vi "Main_08a.vi"() -> ()   [LabVIEW 2023]
uses:
  Map_Direction.ctl
  Cluster_Right Left.ctl
  <vilib>/Utility/error.llb/Trim Whitespace One-Sided.vi
panel:
  out "Map":T1
  in  "Example 2":string="LLR\n\nAAA = (BBB, BBB)\nBBB = (AAA, ZZZ)\nZZZ = (ZZZ, ZZZ)"
  out "Answer":i32
  in  "Puzzle":string="LRRLRRLRRRLRLLRRRLLRRRLRLRRRLRLRRLRRRLRRRLRLRRRLRRRLRRLRRRLLLRLRRRLRRRLRRRLRLRLRRLLRRRLRLLRLRRRLRRLLRLRLRRLRRRLRRLLRLRRRLLRRLRRRLRLRRLLRRRLRRLLRRLRRRLRLRRRLRRLRRRLRRRLRRLRRRLRLRRLRRRLRRRLRRLLRLRRLRRLRRRLRLLLRRRLLRRRLRLRRRLRLRRLRRRLLLRLRRRLRLRRLRRRLRRRLRRLRLRLRRRR\n\nPBN = (JRP, RVT)\nXRS = (CRH, SXK)\nMLN = (STJ, MGB)\nXGX = (XGM, GKP)\nVDC = (DBF, FVR)\nNBC = (QQJ, XKG)\nKRC = (QVQ, RJL)\nLCX = (CSN, DBP)\nMSX = (LVF, PPD)\nMMF = (GBX, LCX)\nBXQ = (MPS, GLM)\nGTL = (VSF, DVZ)\nSVR = (FKK, FJN)\nHJJ = (XPS, HVS)\nMHL = (HTN, HTG)\nLGQ = (NJT, NML)\nKFR = (TXK, DHG)\nMXQ = (DGJ, MKP)\nXST = (MGP, QSK)\nBNJ = (NBC, DFB)\nJLK = (RJS, XDM)\nBKS = (SLF, PLK)\nLCV = (RVB, CJV)\nGJL = (FRB, QNK)\nFPD = (SFN, MLS)\nHMJ = (MXK, CRR)\nSQF = (MCC, QXB)\nCGC = (SCS, FFB)\nCTP = (RJQ, BSV)\nQCF = (JCB, TKP)\nLBJ = (XKV, DQM)\nRMC = (LLD, TTP)\nLHK = (CDB, TSV)\nHPC = (QLX, QPQ)\nVXC = (PLF, SSV)\nRDT = (GJL, TTN)\nSDB = (MVL, FRF)\nHRT = (DVS, BHX)\nMHR = (VXR, VQN)\nRPT = (BLP, DDP)\nJFF = (DCJ, XST)\nNDL = (NJQ, BNC)\nFXL = (MSC, JSR)\nDVZ = (JVJ, KLP)\nXGD = (RFH, DTL)\nMPR = (QNN, CKH)\nSBB = (VTK, TSS)\nDRJ = (GHM, NFK)\nLXL = (SSJ, CQR)\nBTN = (MXN, HLF)\nSMX = (VFT, NKJ)\nRJQ = (STS, GLR)\nQLV = (PNP, TDK)\nQMJ = (MKP, DGJ)\nXDM = (SFB, JLN)\nLFX = (CDM, LMX)\nQTX = (RVB, CJV)\nCPX = (TTH, CBK)\nTFF = (CLG, LGN)\nJDC = (BHH, HFJ)\nTXV = (JVF, FXS)\nLBP = (PRS, PRS)\nLND = (QLV, TLK)\nRXR = (BVT, QKX)\nRSR = (GFN, GVL)\nFLG = (RMC, LTD)\nTPB = (PJP, QCL)\nKQH = (LRG, MRL)\nVVN = (KPP, HJH)\nNTR = (RPQ, GFG)\nQDK = (JFC, XGN)\nVBA = (KLP, JVJ)\nXSP = (KVF, VJV)\nHVB = (CQR, SSJ)\nXBN = (GBD, TCS)\nRFH = (FGN, NSP)\nHTN = (NBH, SMP)\nPSD = (FLS, KCJ)\nMGB = (SDF, MHR)\nNXT = (HKQ, MLD)\nMHC = (JSR, MSC)\nKPP = (HHV, FNC)\nTSS = (RBD, LGQ)\nBMS = (NLL, NFJ)\nBKV = (NLK, BBH)\nSDF = (VXR, VQN)\nGLR = (LFX, XXL)\nNBN = (SXB, DLD)\nCVV = (KGX, DTQ)\nVKG = (VNG, PTR)\nFJR = (KNQ, XGX)\nRJN = (PGR, QCV)\nCNJ = (LSV, BVN)\nDTC = (RXR, MHX)\nFVB = (BSM, BGR)\nSFG = (KSP, GXM)\nPLN = (PDV, XJD)\nTHL = (KRC, HXH)\nPNP = (JQQ, SMV)\nSTS = (LFX, XXL)\nNNC = (MPG, RVG)\nNJT = (JGJ, CGH)\nSCS = (NSR, DXX)\nGSF = (LHP, FTK)\nGBD = (DSN, HRT)\nJVF = (HPT, QHF)\nPSV = (NJC, CPH)\nJLP = (FGD, BFF)\nCRR = (PRB, HCH)\nFVJ = (VBP, BBQ)\nMVL = (CGS, BFN)\nJXK = (SFN, MLS)\nSSV = (DJB, TRK)\nLXQ = (LSB, SPC)\nLHS = (SSV, PLF)\nDDK = (QXR, QCF)\nXKG = (BTS, KFL)\nTSM = (QCV, PGR)\nCPT = (TMH, DFQ)\nDGJ = (MMD, PJN)\nMQP = (CFG, LRB)\nRQM = (JTK, PLN)\nPLK = (KQF, HSZ)\nHVC = (NLK, BBH)\nLSB = (NDT, TPG)\nRMN = (SKJ, PBH)\nQXL = (JNC, XMH)\nTDD = (BSX, GBR)\nBGP = (LBP, LBP)\nTVA = (FBB, VBN)\nVSB = (VNG, PTR)\nXLH = (HMX, FJX)\nNVQ = (RPQ, RPQ)\nFMN = (BSV, RJQ)\nXMC = (QCD, RJK)\nHPT = (HGL, GNS)\nCMS = (KVT, FQR)\nQHF = (HGL, GNS)\nQNT = (BPT, FLG)\nKVD = (SLL, GGK)\nDMK = (HKT, CGD)\nCRM = (BTR, GHV)\nTPJ = (GCT, DQD)\nKFL = (RDG, VDC)\nQCR = (DNK, THD)\nCLV = (MTS, PBN)\nZZZ = (DPM, TCG)\nQHN = (TNC, KVD)\nNRP = (SQL, PMR)\nJNH = (TKD, LQF)\nVPR = (PKX, CTD)\nLVD = (MQC, QKJ)\nXRM = (BRM, MPR)\nFFB = (NSR, DXX)\nMGR = (MNB, TSP)\nFMK = (THR, VGR)\nKVT = (GSN, RXF)\nVMS = (LPM, VJP)\nDVA = (MHC, FXL)\nMXS = (RJS, XDM)\nKXV = (KPF, NKX)\nBBH = (XSP, GMD)\nPKX = (XHC, CPV)\nNSL = (SMX, DNM)\nDXV = (LPM, VJP)\nCCC = (LCX, GBX)\nJVS = (HJJ, FLF)\nHPM = (QSF, CPT)\nFVS = (XXR, CGF)\nPPB = (XGX, KNQ)\nXPF = (SMX, DNM)\nHLF = (NQJ, CVV)\nTJS = (LXQ, VFB)\nFJK = (FGD, BFF)\nQGQ = (FVJ, BDV)\nGRR = (JKM, JLH)\nGHV = (XGD, QBH)\nRVT = (PVB, PCS)\nTBL = (VGK, KTT)\nSNR = (GCT, DQD)\nXSK = (BLL, MNF)\nVDS = (CCC, MMF)\nRVG = (XSK, XSJ)\nTKP = (MLN, KRX)\nSRP = (QLV, TLK)\nFXQ = (LVD, RHD)\nLVC = (LCT, LKS)\nHNC = (MQP, KTG)\nDFP = (NMX, JFX)\nJVT = (SNX, KQK)\nJSR = (KXN, LXS)\nHCV = (MFD, KJX)\nRBJ = (JKT, HLZ)\nHFC = (JFX, NMX)\nXQG = (PGD, XFT)\nFRB = (HCP, LVJ)\nLQF = (QCR, XTL)\nVGR = (RMN, LNQ)\nMMN = (HDR, JTL)\nPJN = (VNM, KHQ)\nTRK = (NSL, XPF)\nTVG = (CJH, THL)\nDMH = (GPM, MSX)\nVTK = (RBD, LGQ)\nTMH = (BSQ, CMT)\nJPN = (LTH, LST)\nSFB = (NKN, RFM)\nCGD = (VBH, ZZZ)\nVNM = (LMT, VRQ)\nNNT = (HHX, NTF)\nVFQ = (HMJ, VFV)\nSQL = (BCQ, NBN)\nQKJ = (GHN, HCK)\nMMR = (KMF, HPM)\nPFS = (HVL, CTG)\nFVD = (LBJ, DVM)\nSLF = (KQF, KQF)\nBBQ = (RSV, LHK)\nTCG = (NGG, LLS)\nBLR = (PTL, MSR)\nCVH = (MVL, FRF)\nGHN = (CKF, HTV)\nXQC = (QXR, QCF)\nGCT = (BGP, BGP)\nXMJ = (BVN, LSV)\nLBH = (VQX, SBC)\nBNC = (LNH, CRM)\nTHP = (KBC, MHH)\nVRQ = (VVN, THX)\nBFN = (SGD, QXL)\nTFH = (TDD, HGV)\nMLS = (PRJ, JPQ)\nXDQ = (BXQ, RQR)\nDJS = (MTS, PBN)\nSSK = (HKQ, MLD)\nVBH = (TCG, DPM)\nNNJ = (JHS, KFR)\nJRP = (PCS, PVB)\nFDK = (SRP, LND)\nFCL = (HPC, NGH)\nBGR = (MFV, CXJ)\nHDR = (FXQ, KSN)\nPPD = (PKL, KTR)\nBLP = (DKJ, DKJ)\nBCX = (PTL, MSR)\nFLF = (HVS, XPS)\nJPQ = (DMH, RTN)\nGNS = (SLT, HHM)\nGVH = (PRS, XKZ)\nPDV = (VDK, VDK)\nPQF = (BQN, CHK)\nSCX = (NLL, NFJ)\nJNC = (VNN, FVD)\nTHR = (LNQ, RMN)\nVBP = (RSV, LHK)\nMTS = (JRP, RVT)\nNKG = (RPG, TFH)\nLXK = (JXM, GSF)\nTXK = (RJC, QNT)\nSMV = (FTJ, GPD)\nDCP = (FFB, SCS)\nCJK = (FJR, PPB)\nLGN = (NLF, MTJ)\nCKF = (SMF, BSH)\nTRP = (TNC, KVD)\nTPG = (DJM, XMK)\nVJC = (JSX, NBT)\nLFK = (RXR, MHX)\nSBX = (FJN, FKK)\nFBB = (BMS, SCX)\nBHX = (SDN, HTF)\nCSN = (NHV, QVH)\nQQJ = (BTS, KFL)\nHFJ = (MMR, KCR)\nSVS = (GFN, GVL)\nFJL = (CJJ, GQF)\nDHG = (QNT, RJC)\nPCS = (VFG, SQF)\nRVB = (SBB, TND)\nPVB = (SQF, VFG)\nLPJ = (LRK, LXK)\nGVL = (NGL, GNV)\nCTJ = (QCD, RJK)\nPQB = (HMD, TQB)\nMCC = (SFV, DVV)\nQXX = (VBC, QGQ)\nRNM = (XXQ, LLT)\nHXB = (TRP, QHN)\nJFC = (TFF, DFC)\nSQQ = (JQL, HNC)\nKHQ = (LMT, VRQ)\nXCC = (FMK, DGK)\nJTL = (FXQ, KSN)\nNLF = (MLK, PLD)\nFVR = (GVK, CMS)\nSMF = (SNR, TPJ)\nNJL = (TRP, QHN)\nCSR = (DVP, KHX)\nQNJ = (THL, CJH)\nSBT = (XST, DCJ)\nRLX = (DGK, FMK)\nTHX = (KPP, HJH)\nKTG = (CFG, LRB)\nPVC = (RQR, BXQ)\nDLD = (GSM, DTT)\nBFF = (JBH, JVT)\nQKX = (FQJ, SFJ)\nDQD = (BGP, XHS)\nVFB = (LSB, SPC)\nMSR = (VBK, JTQ)\nCKB = (HHX, NTF)\nFLS = (QNM, PQB)\nQSF = (TMH, DFQ)\nFTK = (FDK, FLQ)\nFJX = (JVC, GXS)\nBDF = (MPR, BRM)\nMXK = (PRB, HCH)\nSDQ = (FJX, HMX)\nJCC = (TSP, MNB)\nGKP = (JLK, MXS)\nMRL = (FVS, NLQ)\nDPM = (LLS, NGG)\nGFL = (DDJ, NKG)\nFBG = (RDT, MVG)\nKJX = (VCJ, GHB)\nGFC = (LLT, XXQ)\nLVJ = (DJS, CLV)\nKNQ = (XGM, GKP)\nNJN = (FLS, KCJ)\nDSS = (KPF, NKX)\nJVC = (FHD, BMQ)\nTVP = (TBL, MVX)\nBQN = (SHT, TPS)\nDFQ = (CMT, BSQ)\nGXS = (FHD, BMQ)\nLRK = (JXM, GSF)\nKGX = (NDL, XDN)\nVTD = (SXK, CRH)\nKHH = (HKT, HKT)\nNTF = (NVQ, NTR)\nKRX = (STJ, MGB)\nSPC = (NDT, TPG)\nDJM = (JPN, TNG)\nTHD = (VFQ, GCC)\nCLG = (NLF, MTJ)\nNKN = (SRT, VHH)\nGGK = (RLX, XCC)\nHHV = (LCV, QTX)\nLRG = (NLQ, FVS)\nGNG = (BDF, XRM)\nFNC = (QTX, LCV)\nMVV = (QDK, LNK)\nQTH = (MSH, XDC)\nMKP = (MMD, PJN)\nVBC = (FVJ, BDV)\nJKT = (FJL, BNB)\nMFV = (SVS, RSR)\nHKX = (CPH, NJC)\nHCH = (BKV, HVC)\nTLK = (TDK, PNP)\nDNK = (GCC, VFQ)\nVXR = (NJV, KLH)\nMPG = (XSJ, XSK)\nJLN = (NKN, RFM)\nLTH = (QQS, TXV)\nFLQ = (LND, SRP)\nSXN = (MHL, MHL)\nCFG = (BXX, NRP)\nNDT = (XMK, DJM)\nTTP = (VPX, SXR)\nQXR = (TKP, JCB)\nTDK = (JQQ, SMV)\nKXN = (NXH, BNJ)\nVPA = (HTN, HTG)\nVHH = (DSG, NCN)\nAAA = (TCG, DPM)\nGHM = (NNC, VKX)\nGPM = (PPD, LVF)\nCGH = (LVC, BMH)\nNJQ = (LNH, CRM)\nDKB = (HPC, NGH)\nVKB = (KBC, MHH)\nCKH = (LXL, HVB)\nTSP = (BNN, CBJ)\nFKS = (JTK, PLN)\nNGH = (QLX, QPQ)\nMFT = (QMR, CDQ)\nBSV = (GLR, STS)\nRQR = (GLM, MPS)\nDDP = (DKJ, GTL)\nSQP = (MVG, RDT)\nLMX = (PLH, DDV)\nJCB = (KRX, MLN)\nHCP = (DJS, CLV)\nKQF = (MHC, FXL)\nNML = (CGH, JGJ)\nDRG = (KFR, JHS)\nNLQ = (XXR, CGF)\nBNB = (CJJ, GQF)\nMNF = (SQH, HCV)\nHTF = (FHL, FTC)\nJKM = (QNJ, TVG)\nCDM = (DDV, PLH)\nJHS = (TXK, DHG)\nBDK = (TTH, CBK)\nQVQ = (XJC, MFT)\nMMD = (VNM, KHQ)\nRFC = (HVL, CTG)\nBNN = (FGS, SFG)\nQCL = (GFL, KKH)\nKSN = (RHD, LVD)\nXMN = (XQC, DDK)\nNJC = (TSM, RJN)\nSQH = (MFD, KJX)\nQCD = (KHH, KHH)\nKTT = (PSV, HKX)\nSRT = (NCN, DSG)\nMHX = (QKX, BVT)\nCBJ = (FGS, SFG)\nTTH = (TMF, FPL)\nDBF = (GVK, CMS)\nDNM = (NKJ, VFT)\nXGM = (MXS, JLK)\nNLL = (FMJ, CPM)\nHMD = (FKS, RQM)\nPXT = (JTL, HDR)\nGHB = (GGQ, MVV)\nQCV = (VMS, DXV)\nSBC = (FJK, JLP)\nSGD = (XMH, JNC)\nJQQ = (FTJ, GPD)\nJLH = (TVG, QNJ)\nKPF = (XDQ, PVC)\nVQX = (JLP, FJK)\nVDK = (SLF, SLF)\nPLH = (SBX, SVR)\nQNN = (LXL, HVB)\nSXB = (GSM, DTT)\nJQL = (MQP, KTG)\nJXM = (LHP, FTK)\nQXB = (SFV, DVV)\nVBK = (BDK, CPX)\nBVT = (FQJ, SFJ)\nBHK = (KXV, DSS)\nCJJ = (MXQ, QMJ)\nXTL = (DNK, THD)\nBDV = (BBQ, VBP)\nCPH = (RJN, TSM)\nDTA = (FJL, BNB)\nTQB = (FKS, RQM)\nKMR = (NNT, CKB)\nLRB = (BXX, NRP)\nMVG = (TTN, GJL)\nXXL = (LMX, CDM)\nLMT = (VVN, THX)\nQMR = (PFS, RFC)\nBKD = (DVP, KHX)\nQNK = (LVJ, HCP)\nDGK = (THR, VGR)\nXHC = (FBG, SQP)\nTNC = (GGK, SLL)\nVJP = (GGM, HJD)\nVQN = (NJV, KLH)\nLLD = (SXR, VPX)\nXDC = (CST, BHK)\nKQK = (CNJ, XMJ)\nXJC = (QMR, CDQ)\nKKH = (NKG, DDJ)\nFRF = (CGS, BFN)\nFGS = (KSP, GXM)\nGSB = (GBK, VDS)\nNKX = (XDQ, PVC)\nSDN = (FHL, FTC)\nBVN = (CTP, FMN)\nQSK = (DCB, KSC)\nCTD = (CPV, XHC)\nNBH = (XBN, NVB)\nHRS = (LGD, VSK)\nJTQ = (CPX, BDK)\nCMT = (HXP, KMR)\nDKJ = (VSF, VSF)\nVNG = (KQH, PCC)\nCPV = (SQP, FBG)\nNBT = (HJK, GNG)\nVCJ = (GGQ, MVV)\nLNQ = (SKJ, PBH)\nDFB = (QQJ, XKG)\nRJC = (FLG, BPT)\nSFV = (XMN, QJS)\nRHD = (MQC, QKJ)\nQQS = (JVF, FXS)\nNHV = (BMN, GRR)\nNGG = (SQQ, CQQ)\nXGN = (TFF, DFC)\nHCK = (CKF, HTV)\nSNX = (CNJ, XMJ)\nPRB = (HVC, BKV)\nSXR = (SSK, NXT)\nGGQ = (LNK, QDK)\nDCJ = (QSK, MGP)\nMFD = (GHB, VCJ)\nGLM = (XQG, PDF)\nTND = (TSS, VTK)\nJFB = (BLP, BLP)\nKSC = (VKB, THP)\nCXJ = (SVS, RSR)\nVMT = (MXN, HLF)\nNSP = (HCC, TVP)\nBSK = (PKX, CTD)\nMPS = (XQG, PDF)\nNJV = (CJK, MKD)\nCGF = (CGC, DCP)\nGMD = (VJV, KVF)\nCRL = (PJP, QCL)\nMGP = (KSC, DCB)\nCQQ = (JQL, HNC)\nGGZ = (HTG, HTN)\nTNG = (LST, LTH)\nCST = (KXV, DSS)\nVFV = (CRR, MXK)\nRPG = (TDD, HGV)\nCQR = (DRG, NNJ)\nKSP = (DPT, GSB)\nVKX = (MPG, RVG)\nFMJ = (PQF, CVL)\nSLL = (RLX, XCC)\nHLZ = (BNB, FJL)\nGXM = (GSB, DPT)\nBSH = (SNR, TPJ)\nHGL = (HHM, SLT)\nQVH = (GRR, BMN)\nBTR = (XGD, QBH)\nRBD = (NML, NJT)\nHXP = (NNT, CKB)\nBMP = (JCC, MGR)\nKLP = (FGF, TJS)\nNRK = (VBC, QGQ)\nXMK = (TNG, JPN)\nPBH = (GCL, LPJ)\nNSR = (JFB, RPT)\nSHT = (JVS, HKN)\nNVB = (GBD, TCS)\nMLK = (QTH, GTT)\nFTC = (BSK, VPR)\nPCC = (MRL, LRG)\nPTL = (VBK, JTQ)\nNKJ = (FCL, DKB)\nGFN = (NGL, NGL)\nMQC = (GHN, HCK)\nKMF = (QSF, CPT)\nDDV = (SBX, SVR)\nKHX = (BLR, BCX)\nDVP = (BCX, BLR)\nKBC = (MCG, FKC)\nFJN = (JFF, SBT)\nFKK = (JFF, SBT)\nDDJ = (RPG, TFH)\nJVM = (JCC, MGR)\nPJH = (JKT, JKT)\nGNV = (SXN, KFC)\nLKS = (CVH, SDB)\nJBH = (SNX, KQK)\nXSJ = (MNF, BLL)\nMNB = (BNN, CBJ)\nFQR = (RXF, GSN)\nNCN = (LHS, VXC)\nXXR = (DCP, CGC)\nTSQ = (BSM, BGR)\nVSK = (BMP, JVM)\nDTQ = (XDN, NDL)\nLSV = (FMN, CTP)\nFHD = (NJL, HXB)\nMTJ = (PLD, MLK)\nLBC = (CSR, BKD)\nNGL = (SXN, SXN)\nDSN = (BHX, DVS)\nLLT = (VJC, DSF)\nXJD = (VDK, BKS)\nHGV = (BSX, GBR)\nHKT = (VBH, VBH)\nFGN = (HCC, TVP)\nHHG = (CSR, BKD)\nTSV = (HFC, DFP)\nFBK = (TSQ, FVB)\nFGD = (JVT, JBH)\nCGS = (SGD, QXL)\nSLT = (HHG, LBC)\nHMX = (JVC, GXS)\nBVG = (VSK, LGD)\nGSM = (FPD, JXK)\nRJK = (KHH, DMK)\nLNH = (GHV, BTR)\nPLF = (DJB, TRK)\nPMR = (NBN, BCQ)\nCDB = (HFC, DFP)\nHSZ = (FXL, MHC)\nFHL = (BSK, VPR)\nJTK = (PDV, XJD)\nMVX = (KTT, VGK)\nGPD = (JNH, JDV)\nJGJ = (BMH, LVC)\nJVJ = (TJS, FGF)\nCVL = (BQN, CHK)\nSSJ = (NNJ, DRG)\nJDV = (TKD, LQF)\nJFX = (PSD, NJN)\nRXF = (TKS, LBH)\nCDQ = (PFS, RFC)\nFKC = (NRK, QXX)\nBMH = (LKS, LCT)\nMSH = (BHK, CST)\nLLS = (CQQ, SQQ)\nLST = (QQS, TXV)\nGSN = (LBH, TKS)\nRSV = (TSV, CDB)\nDJB = (XPF, NSL)\nGBR = (DTC, LFK)\nMKD = (FJR, PPB)\nHHX = (NVQ, NTR)\nLTD = (TTP, LLD)\nHKQ = (CTJ, XMC)\nKTR = (RNM, GFC)\nNMX = (NJN, PSD)\nFFP = (HFJ, BHH)\nBTS = (VDC, RDG)\nGBK = (MMF, CCC)\nMCG = (NRK, QXX)\nLCT = (CVH, SDB)\nCTG = (XRS, VTD)\nVJV = (BTN, VMT)\nHHM = (LBC, HHG)\nNQJ = (DTQ, KGX)\nMLD = (CTJ, XMC)\nBSM = (CXJ, MFV)\nGQF = (QMJ, MXQ)\nDXX = (JFB, RPT)\nBRM = (CKH, QNN)\nTKS = (SBC, VQX)\nKCR = (KMF, HPM)\nFGF = (VFB, LXQ)\nGFG = (PJH, RBJ)\nXXQ = (DSF, VJC)\nTKD = (QCR, XTL)\nKVF = (BTN, VMT)\nKCJ = (PQB, QNM)\nVSF = (KLP, JVJ)\nSKJ = (GCL, LPJ)\nDBP = (QVH, NHV)\nJSX = (GNG, HJK)\nDSF = (JSX, NBT)\nPLD = (QTH, GTT)\nCJT = (NFK, GHM)\nNFK = (VKX, NNC)\nHTV = (SMF, BSH)\nDTL = (NSP, FGN)\nQPQ = (TPB, CRL)\nDVM = (XKV, DQM)\nSXK = (VSB, VKG)\nPJP = (GFL, KKH)\nDSG = (LHS, VXC)\nCPM = (CVL, PQF)\nSTJ = (SDF, MHR)\nXDN = (NJQ, BNC)\nPRS = (FBB, VBN)\nCJH = (KRC, HXH)\nBHH = (KCR, MMR)\nGCC = (VFV, HMJ)\nRFM = (SRT, VHH)\nPGR = (VMS, DXV)\nSMP = (NVB, XBN)\nPKL = (GFC, RNM)\nPDF = (PGD, XFT)\nDPT = (VDS, GBK)\nBXX = (SQL, PMR)\nDFC = (CLG, LGN)\nGCL = (LRK, LXK)\nBMQ = (HXB, NJL)\nXPS = (XLH, SDQ)\nCHK = (TPS, SHT)\nDCB = (VKB, THP)\nPTR = (KQH, PCC)\nRJL = (XJC, MFT)\nMHH = (MCG, FKC)\nPRJ = (DMH, RTN)\nCBK = (TMF, FPL)\nNLK = (XSP, GMD)\nFPL = (HRS, BVG)\nHCC = (MVX, TBL)\nGTT = (XDC, MSH)\nVNN = (DVM, LBJ)\nPGD = (FFP, JDC)\nLVF = (PKL, KTR)\nLHP = (FLQ, FDK)\nGVK = (KVT, FQR)\nKLH = (CJK, MKD)\nBMN = (JKM, JLH)\nLXS = (BNJ, NXH)\nVFT = (FCL, DKB)\nLPM = (HJD, GGM)\nQLX = (CRL, TPB)\nFXS = (QHF, HPT)\nGBX = (CSN, DBP)\nBCQ = (DLD, SXB)\nHTG = (NBH, SMP)\nDVS = (HTF, SDN)\nXMH = (FVD, VNN)\nBLL = (HCV, SQH)\nQBH = (RFH, DTL)\nFQJ = (FBK, MMT)\nCRH = (VKG, VSB)\nMSC = (LXS, KXN)\nHJD = (MMN, PXT)\nLGD = (BMP, JVM)\nDVV = (XMN, QJS)\nNFJ = (FMJ, CPM)\nMXN = (NQJ, CVV)\nVFG = (MCC, QXB)\nTCS = (DSN, HRT)\nBSQ = (HXP, KMR)\nHVS = (SDQ, XLH)\nMMT = (FVB, TSQ)\nXHS = (LBP, GVH)\nHXH = (RJL, QVQ)\nDTT = (JXK, FPD)\nHJH = (HHV, FNC)\nQNM = (TQB, HMD)\nRPQ = (PJH, PJH)\nDQM = (DRJ, CJT)\nRJS = (JLN, SFB)\nNXH = (DFB, NBC)\nGGM = (MMN, PXT)\nFTJ = (JDV, JNH)\nBSX = (DTC, LFK)\nHKN = (FLF, HJJ)\nVGK = (HKX, PSV)\nVPX = (NXT, SSK)\nSFJ = (MMT, FBK)\nKFC = (MHL, GGZ)\nRDG = (DBF, FVR)\nRTN = (MSX, GPM)\nQJS = (XQC, DDK)\nXKZ = (VBN, FBB)\nTMF = (HRS, BVG)\nCJV = (TND, SBB)\nXFT = (JDC, FFP)\nTPS = (HKN, JVS)\nBPT = (RMC, LTD)\nHVL = (XRS, VTD)\nHJK = (XRM, BDF)\nXKV = (CJT, DRJ)\nSFN = (JPQ, PRJ)\nTTN = (QNK, FRB)\nLNK = (XGN, JFC)\nVBN = (BMS, SCX)"
  in  "Example":string="RL\n\nAAA = (BBB, CCC)\nBBB = (DDD, EEE)\nCCC = (ZZZ, GGG)\nDDD = (DDD, DDD)\nEEE = (EEE, EEE)\nGGG = (GGG, GGG)\nZZZ = (ZZZ, ZZZ)"
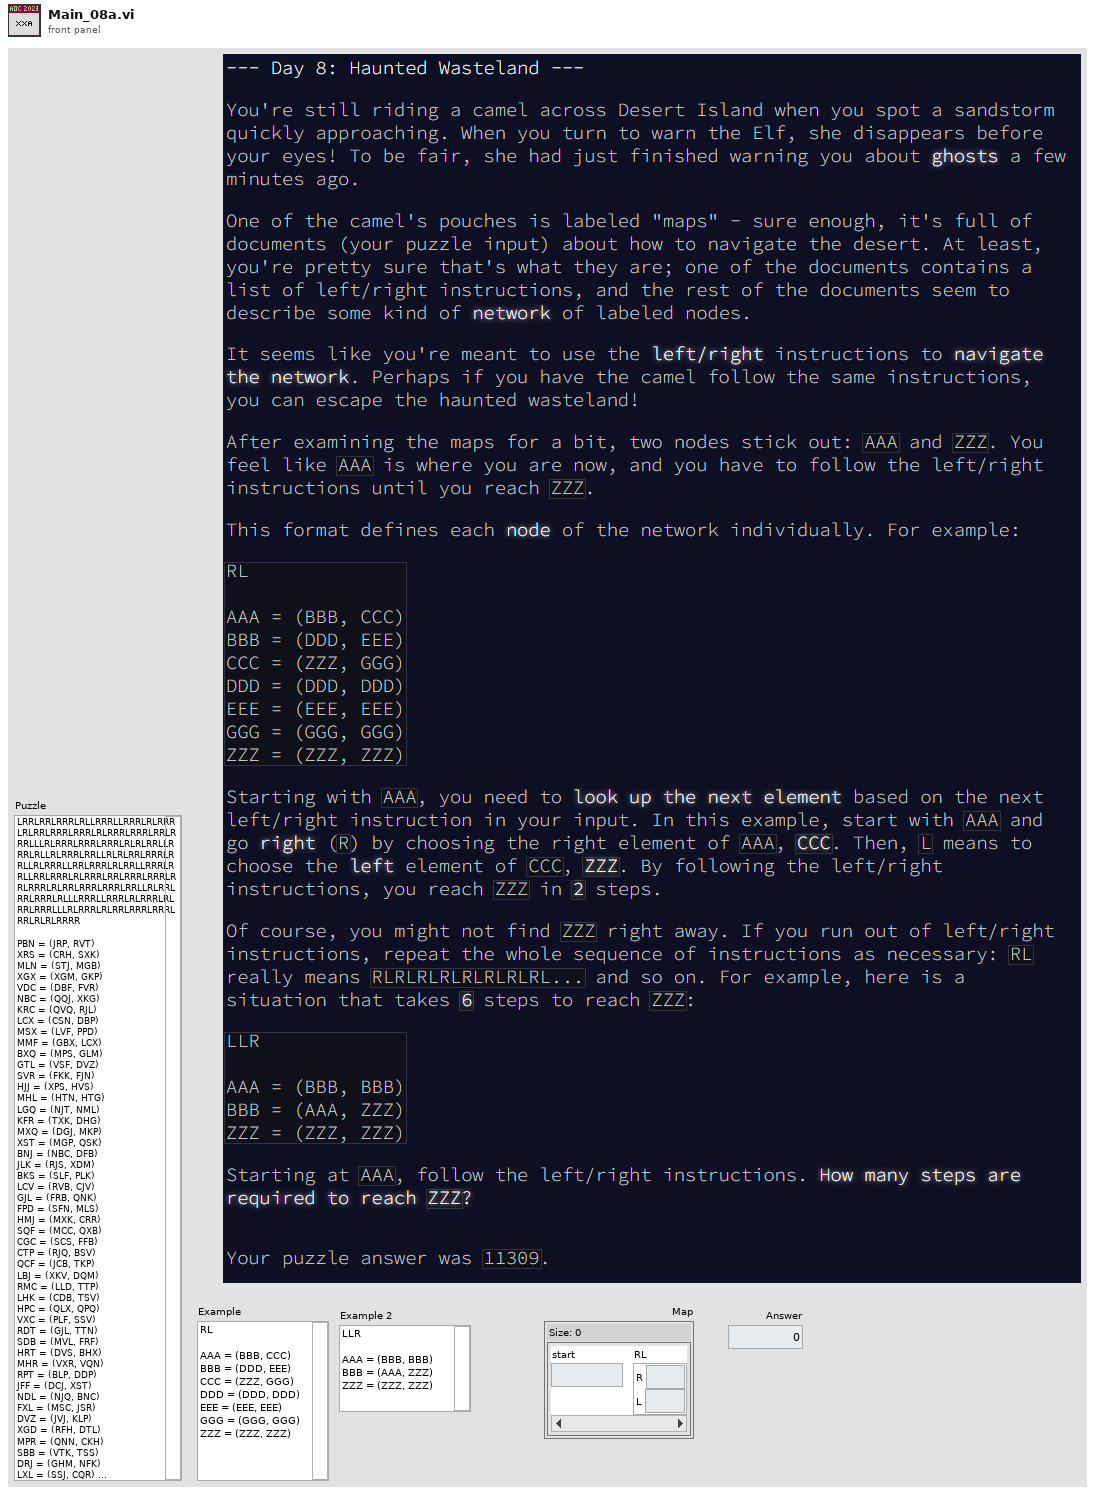
[diagram p1: front panel]
types:
  T1 = typedef "Map_Direction.ctl" = map{string, T2}
  T2 = typedef "Cluster_Right Left.ctl" = cluster{"R":string, "L":string}
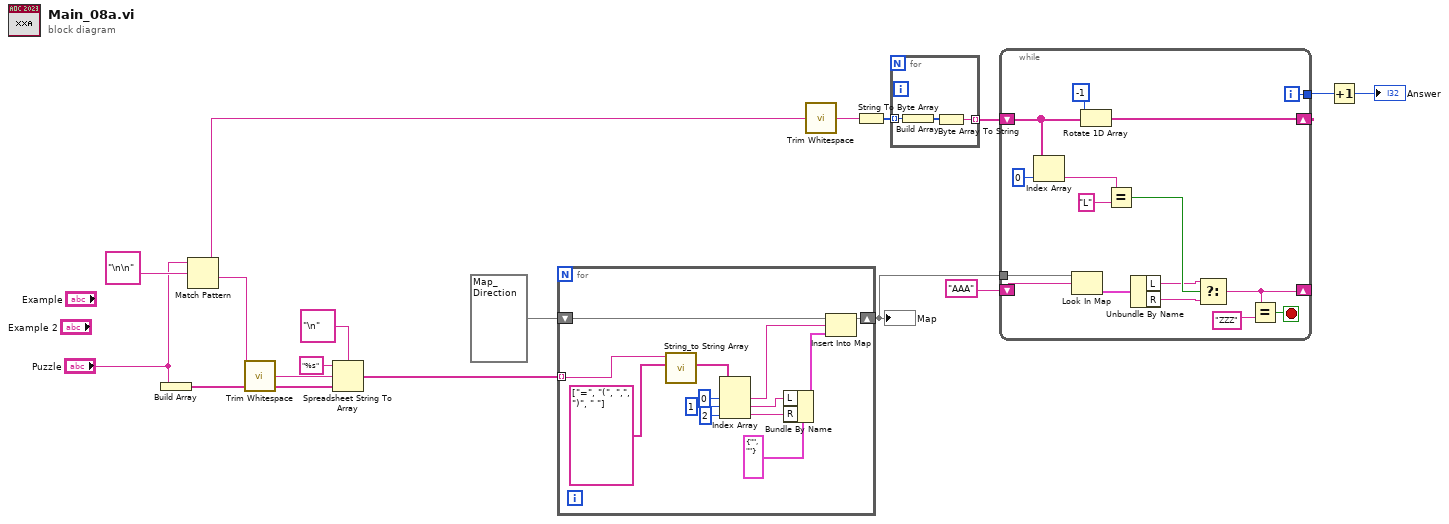
[diagram p0: block diagram]
diagram:
  n1 = Build Array("Puzzle") -> (w17:string[])
  n2 = Match Pattern(string="Puzzle", regular expression="\n\n" ("delimiter (Tab)")) -> (before substring=w12:string, after substring=w13:string)  [unwired: 1 in, 2 out]
  n3 = call <vilib>:"Trim Whitespace.vi"("string"=w13) -> ("trimmed string"=w9:string)  [unwired: 1 in]
  n4 = Spreadsheet String To Array(delimiter (Tab)="\n", format string="%s", spreadsheet string=w9, array type (2D Dbl)=w17) -> (array=w8:string[])
  n5 = for {
    tunnel: w8 -> [w30] mode=indexing
    shift-right: [w23] -> w6
    shift-left: T1 {} ("Map") -> [w24]
    n6 = call "String_to String Array.vi"("Seperators (;)"=string[] ["=", "(", ",", ")", " "], "Input String"=w30) -> ("String Array Out Blanks Removed Out"=w28:string[])  [unwired: 7 in, 2 out]
    n7 = Index Array(array=w28, index #1=0 ("index"), index #2=1 ("index"), index #3=2 ("index")) -> (element #1=w22:string, element #2=w19:string, element #3=w18:string)
    n8 = Bundle By Name(cluster=T2 {"R"="", "L"=""} ("Cluster"), "L"=w19, "R"=w18) -> (w20:T2)
    n9 = Insert Into Map(map in=w24, key=w22, value=w20) -> (map out=w23:T1)  [unwired: 2 out]
  }
  "Map" <- w6
  n10 = call <vilib>:"Trim Whitespace.vi"("string"=w12) -> ("trimmed string"=w10:string)  [unwired: 1 in]
  n11 = String To Byte Array(string=w10) -> (unsigned byte array=w11:u8[])
  n12 = for {
    tunnel: w11 -> [w33] mode=indexing
    tunnel: [w31] -> w5 mode=indexing
    n13 = Build Array(w33) -> (w32:u8[])
    n14 = Byte Array To String(unsigned byte array=w32) -> (string=w31:string)
  }
  n15 = while {
    tunnel: w6 -> [w42]
    shift-right: [w34] -> _
    shift-left: "AAA" -> [w41]
    shift-right: [w43] -> _
    shift-left: w5 -> [w45]
    tunnel: [w47] -> w3
    i -> [w47]
    stop <- w48 stop-if-true
    n16 = Index Array(array=w45, index=0) -> (element=w39:string)
    n17 = Look In Map(map=w42, key=w41) -> (value=w40:T2)  [unwired: 1 in, 1 out]
    n18 = Rotate 1D Array(1:w45, 2:-1 ("n")) -> (0:w43:string[])
    n19 = Equal?(x=w39, y="L") -> (x = y?=w37:bool)
    n20 = Unbundle By Name(w40) -> ("L"=w36:string, "R"=w35:string)
    n21 = Select(t=w36, s=w37, f=w35) -> (s? t:f=w34:string)
    n22 = Equal?(x=w34, y="ZZZ") -> (x = y?=w48:bool)
  }
  n23 = Increment(x=w3) -> (x+1=→"Answer":i32)
